vi "ActionVIOnLoad.vi"(8 "error in (no error)":errorcluster, 11 "Device Item Ref in":T1 format="%.0x") -> (0 "error out":errorcluster, 3 "Device Item Ref out":T1 format="%.0x")   [LabVIEW 2020, in "Routing and Faulting System Explorer.lvlib"]
uses:
  Routing and Faulting System Explorer.lvlib
  <vilib>/NI VeriStand/Custom Device API/Custom Device Item Ref.ctl
  <vilib>/NI VeriStand/Custom Device API/Custom Device API.lvlib
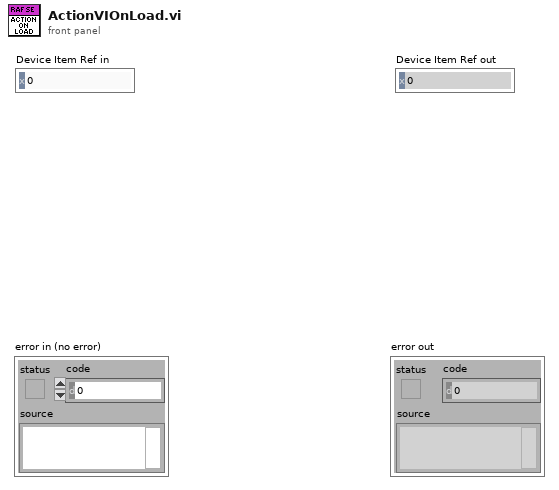
[diagram p1: front panel]
types:
  T1 = typedef "Custom Device API.lvlib/Custom Device Item Ref.ctl" = u64
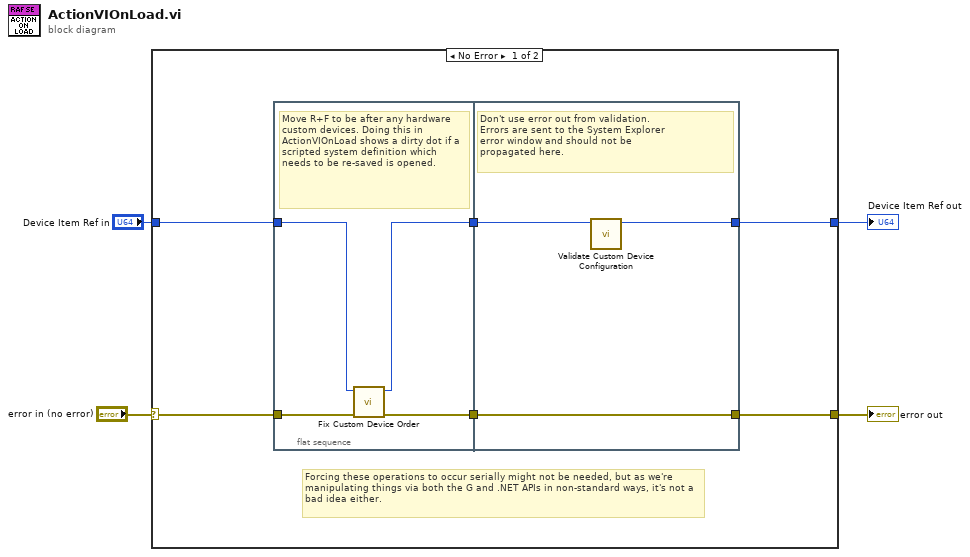
[diagram p0: block diagram]
diagram:
  n1 = case shown="No Error" "error in (no error)" {
    selector: "error in (no error)" -> [w7 w19]
    tunnel: [w8 w19] -> w3
    tunnel: "Device Item Ref in" -> [w10 w18]
    tunnel: [w9 w18] -> w1
    frame No Error {
      # "Forcing these operations to occur serially might not be needed, but as we're manipulating things via both the G and .NET APIs in non-standard ways, it's not a bad idea either."
      n2 = flat-sequence {
        tunnel: w7 -> [w14]
        tunnel: w10 -> [w12]
        tunnel: [w13] -> w6
        tunnel: [w11] -> w5
        tunnel: [w16] -> w9
        tunnel: [w15] -> w8
        tunnel: w6 -> [w15]
        tunnel: w5 -> [w17]
        frame #0 {
          # "Move R+F to be after any hardware custom devices. Doing this in ActionVIOnLoad shows a dirty dot if a scripted system definition which needs to be re-saved is opened."
          n3 = call "Fix Custom Device Order.vi"("error in"=w14, "Device Item Ref in"=w12) -> ("error out"=w13:errorcluster, "Device Item Ref out"=w11:T1)  [unwired: 8 in]
        }
        frame #1 {
          # "Don't use error out from validation.\nErrors are sent to the System Explorer\nerror window and should not be\npropagated here."
          n4 = call "Validate Custom Device Configuration.vi"("Routing and Faulting Custom Device Ref"=w17) -> ("Routing and Faulting Custom Device Ref out"=w16:T1)  [unwired: 8 in, 2 out]
        }
      }
    }
    frame Error {
    }
  }
  "error out" <- w3
  "Device Item Ref out" <- w1
